vi "Set_Time_1.vi"() -> ()   [LabVIEW 2021]
panel:
  out "RT current time":timestamp
  in  "Stop Button":bool
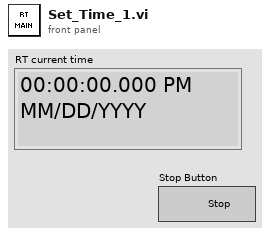
[diagram p1: front panel]
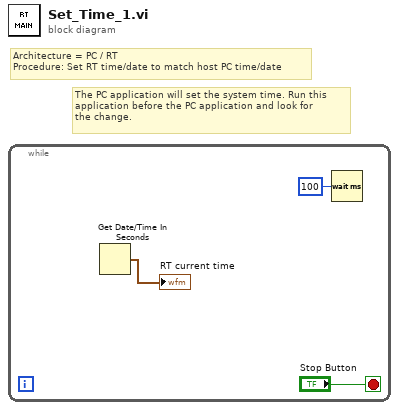
[diagram p0: block diagram]
diagram:
  # "The PC application will set the system time. Run this\napplication before the PC application and look for\nthe change."
  # "Architecture = PC / RT\nProcedure: Set RT time/date to match host PC time/date"
  n1 = while {
    stop <- "Stop Button" stop-if-true
    n2 = Get Date/Time In Seconds() -> (seconds since 1Jan1904=→"RT current time":timestamp)
    n3 = Wait (ms)(milliseconds to wait=u32 100) -> ()  [unwired: 1 out]
  }
